vi "Configure Match Time Timer.vi"(0 "VISA resource name":refnum<visa-resource-name>, 1 "Match Condition - Month (Jan)":u16(ring)=1 items=["Jan"=1, "Feb"=2, "Mar"=3, "Apr"=4, "May"=5, "Jun"=6, "Jul"=7, "Aug"=8, "Sep"=9, "Oct"=10, "Nov"=11, "Dec"=12], 2 "Match Condition - Day (1)":i32=1 min=1 max=31, 3 "Match Condition - Day Of Week (Sun)":u16(ring) items=["Sun", "Mon", "Tue", "Wed", "Thu", "Fri", "Sat"], 5 "Timer No. (1)":i32=1 min=1 max=12, 7 "Type (0: Off)":u16(ring) items=["Off", "Year", "Month", "Week", "Day"], 9 "Timer Action (1: Repeat)":u16(ring)=1 items=["Single", "Repeat"], 11 "error in (no error)":errorcluster, 12 "Match Condition - Hour (1)":i32=1 min=0 max=23, 13 "Match Condition - Minute (1)":i32=1 min=0 max=59) -> (4 "VISA resource name out":refnum<visa-resource-name>, 6 "Timer No.":i32, 15 "error out":errorcluster)   [LabVIEW 2020, in "Yokogawa GX Series.lvlib"]
doc: "Sets a match time timer.\n\nCommand: SMatchTimer"
uses:
  <instrlib>/Yokogawa GX Series/Yokogawa GX Series.lvlib
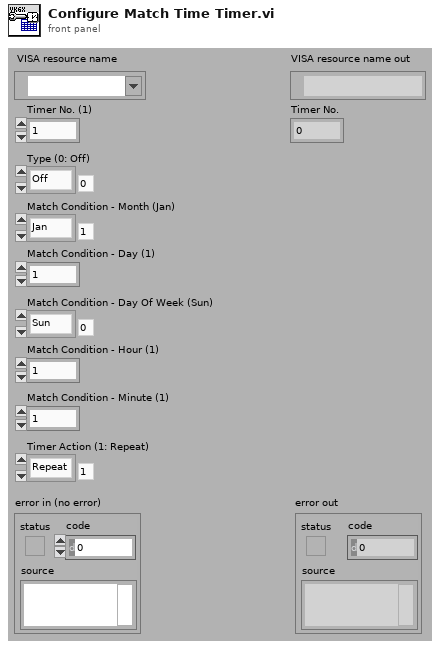
[diagram p1: front panel]
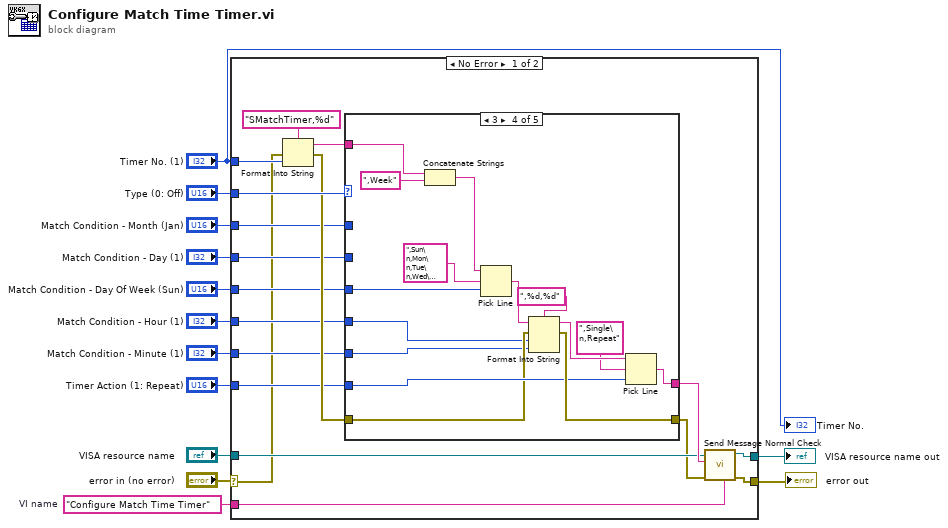
[diagram p0: block diagram]
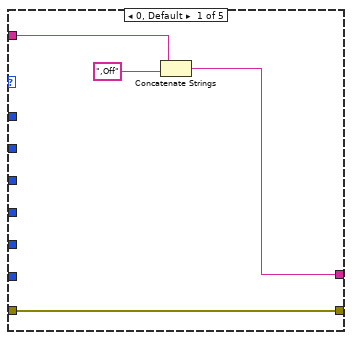
[diagram p2: hidden frame]
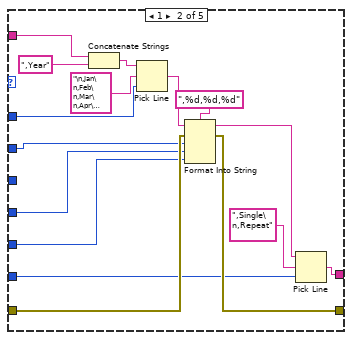
[diagram p3: hidden frame]
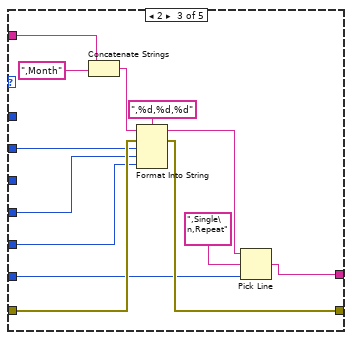
[diagram p4: hidden frame]
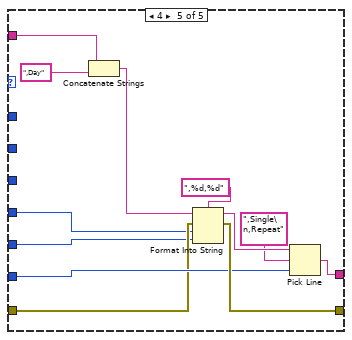
[diagram p5: hidden frame]
diagram:
  w13 = "Configure Match Time Timer"  # VI name
  n1 = case shown="No Error" "error in (no error)" {
    selector: "error in (no error)" -> [w14 w92]
    tunnel: w13 -> [w31 _]
    tunnel: [w30 w93] -> w12
    tunnel: [w29 w92] -> w11
    tunnel: "Type (0: Off)" -> [w27 _]
    tunnel: "VISA resource name" -> [w23 w93]
    tunnel: "Match Condition - Month (Jan)" -> [w21 _]
    tunnel: "Match Condition - Day (1)" -> [w20 _]
    tunnel: "Match Condition - Day Of Week (Sun)" -> [w19 _]
    tunnel: "Match Condition - Hour (1)" -> [w18 _]
    tunnel: "Match Condition - Minute (1)" -> [w17 _]
    tunnel: "Timer Action (1: Repeat)" -> [w16 _]
    tunnel: "Timer No. (1)" -> [w15 _]
    frame No Error {
      n2 = Format Into String(format string="SMatchTimer,%d", error in=w14, w15) -> (resulting string=w25:string, error out=w26:errorcluster)  [unwired: 1 in]
      n3 = case shown="3" w27 {
        tunnel: w26 -> [w32 w47 w61 w71 w83]
        tunnel: w25 -> [w34 w37 w64 w79 w91]
        tunnel: [w33 w39 w52 w72 w84] -> w24
        tunnel: [w32 w46 w59 w76 w88] -> w22
        tunnel: w21 -> [_ w50 _ _ _]
        tunnel: w20 -> [_ w45 w58 _ _]
        tunnel: w19 -> [_ _ _ w65 _]
        tunnel: w18 -> [_ w44 w57 w70 w82]
        tunnel: w17 -> [_ w43 w56 w69 w81]
        tunnel: w16 -> [_ w40 w53 w73 w85]
        frame 0, Default {
          n4 = Concatenate Strings(w34, ",Off") -> (w33:string)
        }
        frame 1 {
          n5 = Concatenate Strings(w37, ",Year") -> (w38:string)
          n6 = Pick Line(string ("")=w38, multi-line string="\n,Jan\n,Feb\n,Mar\n,Apr\n,May\n,Jun\n,Jul\n,Aug\n,Sep\n,Oct\n,Nov\n,Dec", line index=w50) -> (output string=w49:string)
          n7 = Format Into String(format string=",%d,%d,%d", initial string=w49, error in=w47, w45, w44, w43) -> (resulting string=w42:string, error out=w46:errorcluster)
          n8 = Pick Line(string ("")=w42, multi-line string=",Single\n,Repeat", line index=w40) -> (output string=w39:string)
        }
        frame 2 {
          n9 = Concatenate Strings(w64, ",Month") -> (w62:string)
          n10 = Format Into String(format string=",%d,%d,%d", initial string=w62, error in=w61, w58, w57, w56) -> (resulting string=w55:string, error out=w59:errorcluster)
          n11 = Pick Line(string ("")=w55, multi-line string=",Single\n,Repeat", line index=w53) -> (output string=w52:string)
        }
        frame 3 {
          n12 = Concatenate Strings(w79, ",Week") -> (w67:string)
          n13 = Pick Line(string ("")=w67, multi-line string=",Sun\n,Mon\n,Tue\n,Wed\n,Thu\n,Fri\n,Sat", line index=w65) -> (output string=w68:string)
          n14 = Format Into String(format string=",%d,%d", initial string=w68, error in=w71, w70, w69) -> (resulting string=w75:string, error out=w76:errorcluster)
          n15 = Pick Line(string ("")=w75, multi-line string=",Single\n,Repeat", line index=w73) -> (output string=w72:string)
        }
        frame 4 {
          n16 = Concatenate Strings(w91, ",Day") -> (w80:string)
          n17 = Format Into String(format string=",%d,%d", initial string=w80, error in=w83, w82, w81) -> (resulting string=w87:string, error out=w88:errorcluster)
          n18 = Pick Line(string ("")=w87, multi-line string=",Single\n,Repeat", line index=w85) -> (output string=w84:string)
        }
      }
      n19 = call <instrlib>:"Send Message Normal Check.vi"("Source (\"\")"=w31, "error in (no error)"=w22, "Send Message (\"\")"=w24, "VISA resource name"=w23) -> ("error out"=w29:errorcluster, "VISA resource name out"=w30:refnum<visa-resource-name>)  [unwired: 2 in, 4 out]
    }
    frame Error {
    }
  }
  "error out" <- w11
  "VISA resource name out" <- w12
  "Timer No." <- "Timer No. (1)"
